vi "main.vi"() -> ()   [LabVIEW 2024]
panel:
  out "x/y":dbl
  out "x*y":dbl
  out "x-y":dbl
  out "x+y":dbl
  in  "y":dbl
  in  "x":dbl
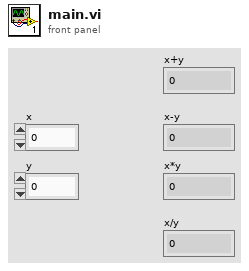
[diagram p1: front panel]
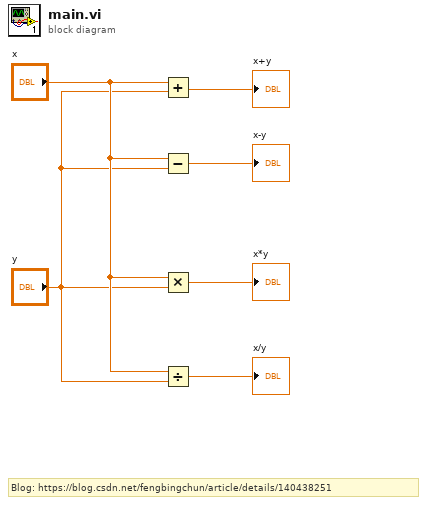
[diagram p0: block diagram]
diagram:
  # "Blog: https://blog.csdn.net/fengbingchun/article/details/140438251"
  n1 = Add(x="x", y="y") -> (x+y=→"x+y":dbl)
  n2 = Subtract(x="x", y="y") -> (x-y=→"x-y":dbl)
  n3 = Multiply(x="x", y="y") -> (x*y=→"x*y":dbl)
  n4 = Divide(x="x", y="y") -> (x/y=→"x/y":dbl)
